vi "GCliWrite.vi"(8 "error in (no error)":errorcluster, 10 "Text to Write":string, 11 "CLI in":refnum<class "CLI.lvclass">) -> (0 "error out":errorcluster, 3 "CLI out":refnum<class "CLI.lvclass">)   [LabVIEW 2023, in "CICD.lvlib"]
uses:
  CICD.lvlib
  <vilib>/Wiresmith Technology/G CLI/CLI Class/CLI.lvclass
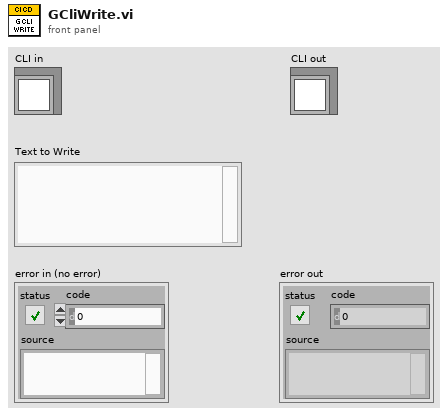
[diagram p1: front panel]
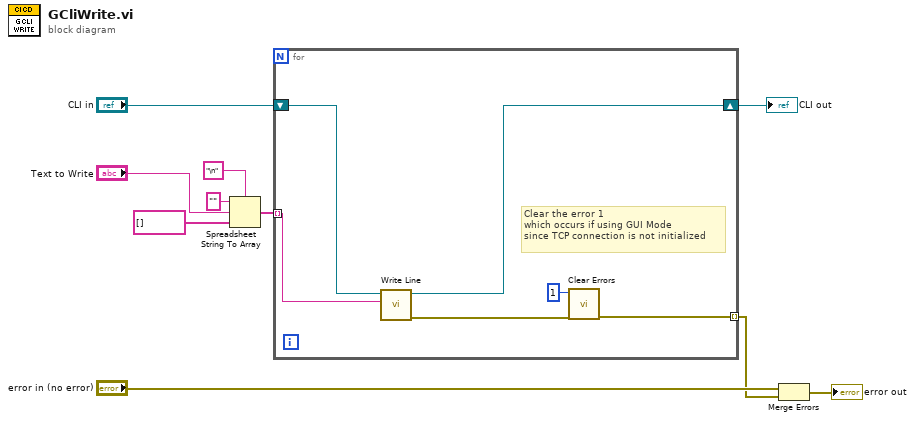
[diagram p0: block diagram]
diagram:
  n1 = Spreadsheet String To Array(delimiter (Tab)="\n", format string="", spreadsheet string="Text to Write", array type (2D Dbl)=string[] []) -> (array=w1:string[])
  n2 = for {
    shift-right: [w16] -> w10
    shift-left: "CLI in" -> [w15]
    tunnel: w1 -> [w11] mode=indexing
    tunnel: [w12] -> w7 mode=indexing
    # "Clear the error 1\nwhich occurs if using GUI Mode\nsince TCP connection is not initialized"
    n3 = call <vilib>:"Write Line.vi"("Text to Write"=w11, "CLI in"=w15) -> ("error out"=w14:errorcluster, "CLI out"=w16:refnum<class "CLI.lvclass">)  [unwired: 8 in]
    n4 = call <vilib>:"Clear Errors.vi"("error in (no error)"=w14, "specific error code to clear (0: all)"=1) -> ("error out"=w12:errorcluster)  [unwired: 4 in, 1 out]
  }
  "CLI out" <- w10
  n5 = Merge Errors("error in (no error)", w7) -> (→"error out":errorcluster)
